vi "Append File to Report.vi"(0 "report in":refnum<class "NI_HTML.lvclass">, 1 "MS Office parameters":T1, 7 "file path":path, 9 "is spreadsheet file? (Excel)":bool, 11 "error in (no error)":errorcluster) -> (4 "report out":refnum<class "NI_HTML.lvclass">, 8 "start out (Word)":i32, 10 "end out (Word)":i32, 15 "error out":errorcluster)   [LabVIEW 2015, in "NI_HTML.lvclass"]
doc: "Appends the text from a text file into the current report."
uses:
  <vilib>/Utility/NIReport.llb/HTML/NI_HTML.lvclass
  <vilib>/Utility/NIReport.llb/HTML/NI_HTML.lvclass/NI_HTML.ctl
  <vilib>/Utility/NIReport.llb/NI_ReportGenerationCore.lvlib
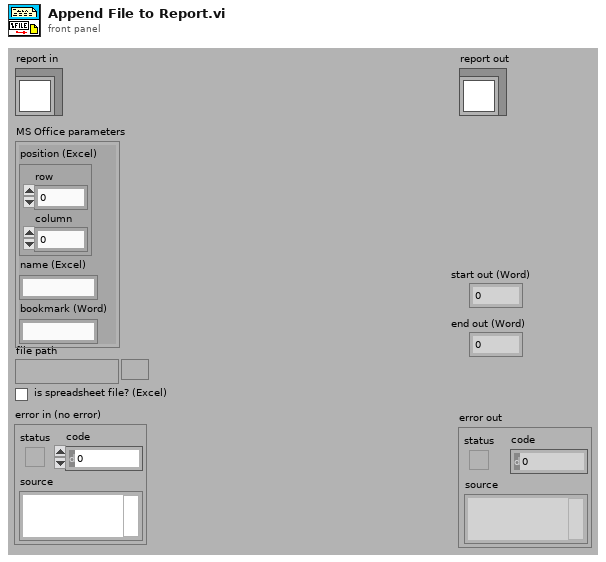
[diagram p1: front panel]
types:
  T1 = cluster{"position (Excel)":cluster{"row":i32, "column":i32}, "name (Excel)":string, "bookmark (Word)":string}
  T2 = typedef "NI_ReportGenerationCore.lvlib/HTML Report Data.ctl" = cluster{"Body Text":string, "Font Tag":string, "Title Text":string, "Header Text":string, "Footer Text":string, "Image List":path[]}
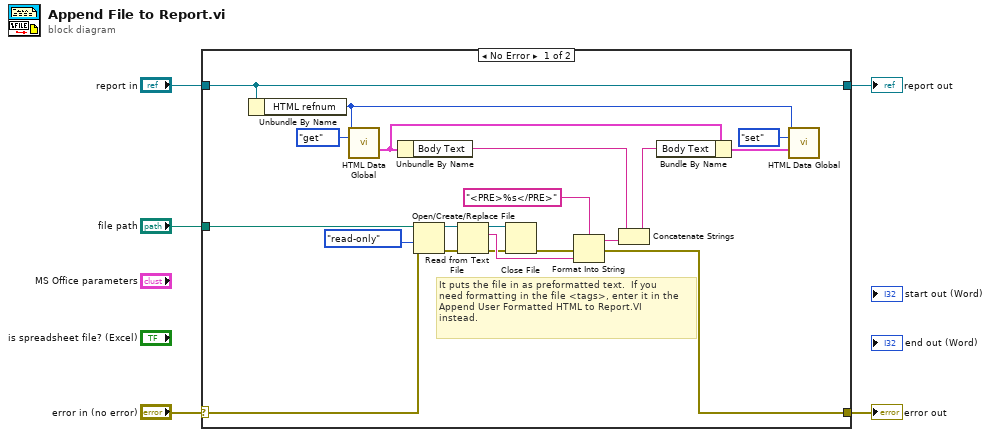
[diagram p0: block diagram]
diagram:
  n1 = case shown="No Error" "error in (no error)" {
    selector: "error in (no error)" -> [w15 w27]
    tunnel: [w14 w27] -> w4
    tunnel: [w11 w26] -> w2
    tunnel: "report in" -> [w11 w26]
    tunnel: "file path" -> [w13 _]
    frame No Error {
      # "It puts the file in as preformatted text.  If you \nneed formatting in the file <tags>, enter it in the \nAppend User Formatted HTML to Report.VI\ninstead."
      n2 = Unbundle By Name(w11) -> ("HTML refnum"=w6:u32)
      n3 = call <vilib>:"HTML Data Global.vi"("HTML refnum"=w6, "menu"=enum16{"init", "get", "set", "delete"}."get") -> ("HTML report data out"=w7:T2)  [unwired: 1 in, 12 out]
      n4 = Unbundle By Name(w7) -> ("Body Text"=w16:string)
      n5 = Open/Create/Replace File(file path (use dialog)=w13, error in=w15, access (0:read/write)=enum16{"read/write", "read-only", "write-only"}."read-only") -> (refnum out=w23:refnum<file>, error out=w22:errorcluster)  [unwired: 4 out]
      n6 = Read from Text File(file (use dialog)=w23, error in=w22) -> (refnum out=w20:refnum<file>, text=w25:string, error out=w19:errorcluster)  [unwired: 3 out]
      n7 = Close File(refnum=w20, error in=w19) -> (error out=w24:errorcluster)  [unwired: 1 out]
      n8 = Format Into String(format string="<PRE>%s</PRE>", error in=w24, w25) -> (resulting string=w18:string, error out=w14:errorcluster)  [unwired: 1 in]
      n9 = Concatenate Strings(w16, w18) -> (w8:string)
      n10 = Bundle By Name(cluster=w7, "Body Text"=w8) -> (w10:T2)
      n11 = call <vilib>:"HTML Data Global.vi"("HTML refnum"=w6, "menu"=enum16{"init", "get", "set", "delete"}."set", "HTML report data in"=w10) -> ()  [unwired: 13 out]
    }
    frame Error {
    }
  }
  "error out" <- w4
  "report out" <- w2
